vi "FSK2.vi"() -> ()   [LabVIEW 2012]
uses:
  <vilib>/express/express analysis/Spectral/Block/exnSpectralBlock spectral measurements peak poly.vi
  <vilib>/express/express analysis/Spectral/Block/exnSpectralBlock spectral measurements peak DDT.vi
  <vilib>/express/express analysis/Spectral/XNode/ExpressSpectralMeasurementsBlockNode.xnode
  <vilib>/measure/NI_MABase.lvlib
panel:
  out "Waveform Chart":i32(graph)
  in  "standard deviation":dbl
  out "Waveform Graph 4":dynamicdata(graph)
  out "Waveform Graph 3":dynamicdata(graph)
  out "Waveform Graph 2":dynamicdata(graph)
  out "Waveform Graph":dynamicdata(graph)
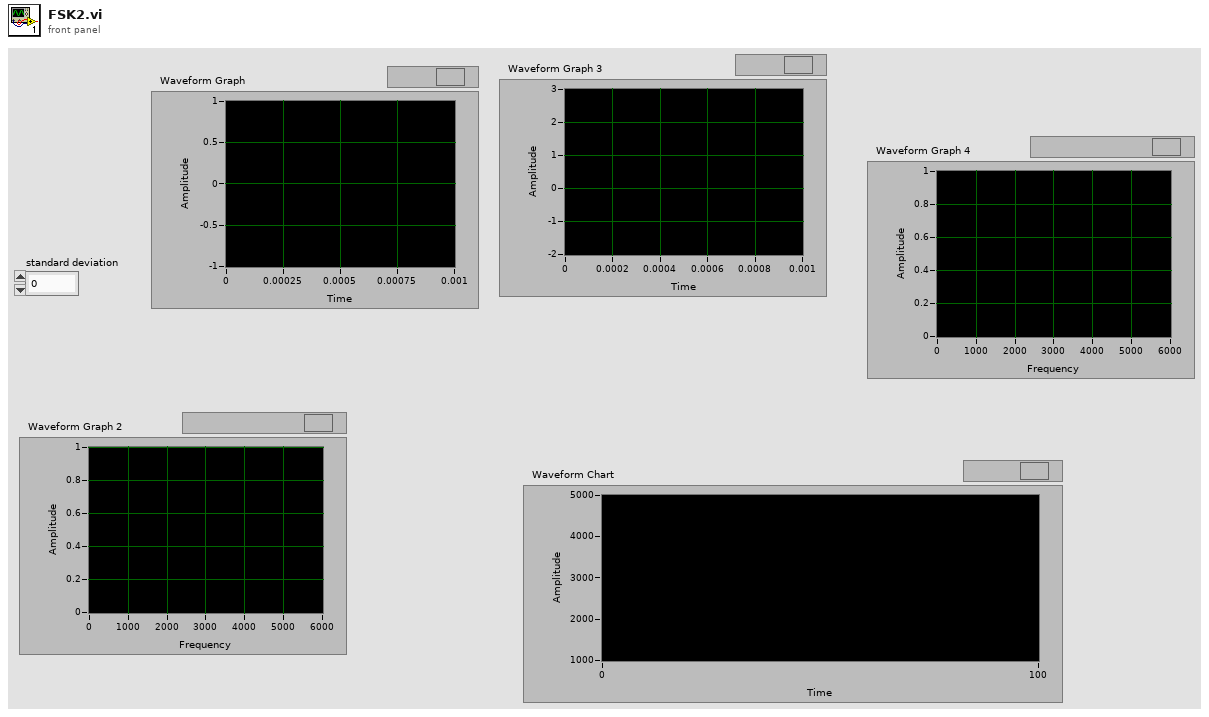
[diagram p1: front panel]
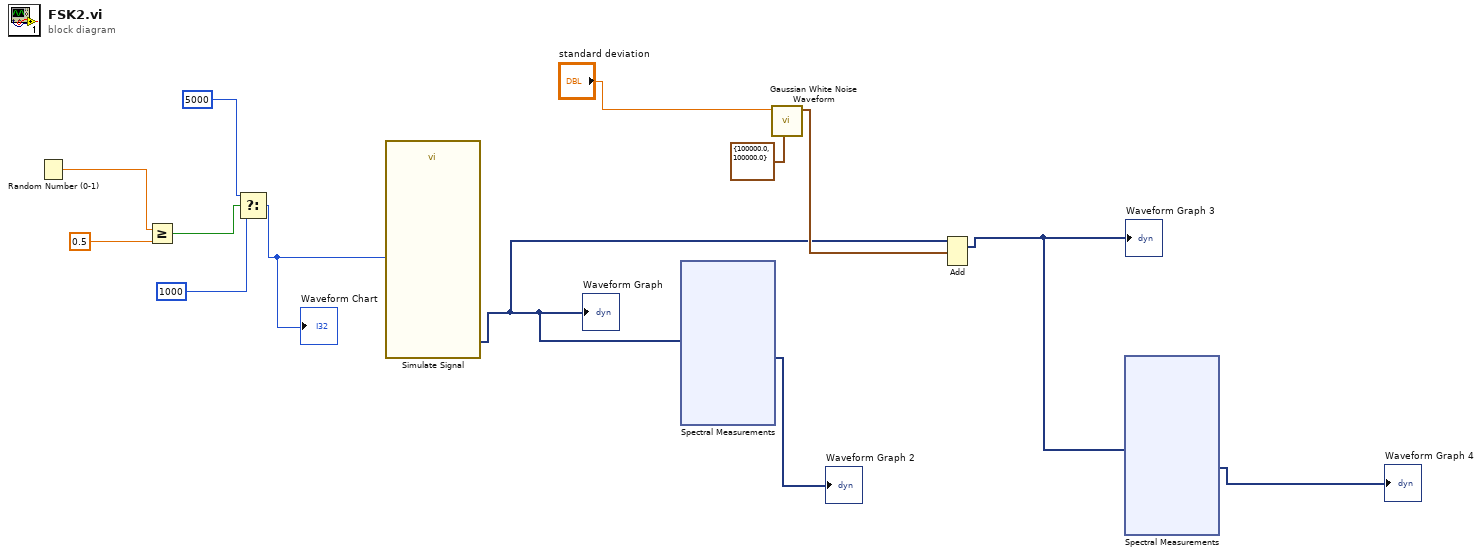
[diagram p0: block diagram]
diagram:
  n1 = Random Number (0-1)() -> (number: 0 to 1=w12:dbl)
  n2 = Greater Or Equal?(x=w12, y=0.5) -> (x >= y?=w13:bool)
  n3 = Select(t=5000, s=w13, f=1000) -> (s? t:f=w1:i32)
  "Waveform Chart" <- w1
  n4 = call "Simulate Signal"("Frequency"=w1) -> ("Sine"=w2:dynamicdata)  [unwired: 13 in, 1 out]
  "Waveform Graph" <- w2
  n5 = xnode "Spectral Measurements"("Signals"=w2) -> ("FFT - (Peak)"=→"Waveform Graph 2":dynamicdata)  [unwired: 1 in, 2 out]
  n6 = call <vilib>:"Gaussian White Noise Waveform.vi"("sampling info"=cluster{"Fs":dbl, "#s":dbl} {"Fs"=100000.0, "#s"=100000.0}, "standard deviation"="standard deviation") -> ("signal out"=w6:waveform(dbl))  [unwired: 8 in, 1 out]
  n7 = Add(1:w6, 2:w2) -> (0:w3:dynamicdata)  [unwired: 1 in, 1 out]
  "Waveform Graph 3" <- w3
  n8 = xnode "Spectral Measurements"("Signals"=w3) -> ("FFT - (Peak)"=→"Waveform Graph 4":dynamicdata)  [unwired: 1 in, 2 out]
